vi "Read.vi"(8 "error in (no error)":errorcluster, 11 "DAQmx AO in":refnum<class "DAQmx AO.lvclass">) -> (0 "error out":errorcluster, 2 "Output":variant, 3 "DAQmx AO out":refnum<class "DAQmx AO.lvclass">)   [LabVIEW 2017, in "DAQmx AO.lvclass"]
uses:
  DAQmx AO.lvclass
  C:/Microcellular Plastics Lab/Hardware Settings/Hardware Types/DAQmx/DAQmx.lvclass
  DAQmx/DAQmx.lvclass/DAQmx.ctl
  <vilib>/DAQmx/read.llb/DAQmx Read (Analog 1D DBL NChan 1Samp).vi
  DAQmx/Accessors/Read DAQmx Task Name.vi
  <vilib>/DAQmx/miscellaneous.llb/DAQmx Fill In Error Info.vi
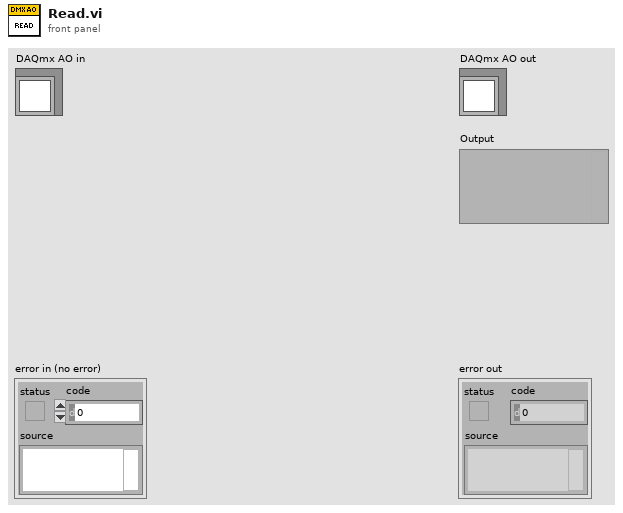
[diagram p1: front panel]
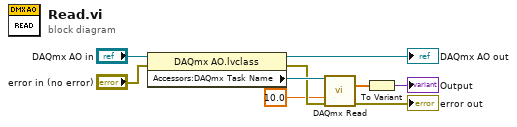
[diagram p0: block diagram]
diagram:
  n1 = property class="DAQmx AO.lvclass"(reference="DAQmx AO in", error in="error in (no error)") -> (reference out=→"DAQmx AO out":refnum<class "DAQmx AO.lvclass">, error out=w2:errorcluster, "Accessors:DAQmx Task Name"=w6:refnum<k21>)
  n2 = call-poly <vilib>:"DAQmx Read.vi"("task/channels in"=w6, "timeout"=10.0, "error in"=w2) -> ("data"=w5:dbl[], "error out"=→"error out":errorcluster)  [unwired: 10 in, 1 out]
  n3 = To Variant(anything=w5) -> (Variant=→"Output":variant)
